vi "SYST_UPR_FPAN_STAT.vi"(0 "VISA IN":refnum<visa-resource-name>, 5 "error in":errorcluster, 7 "Preset":bool) -> (14 "VISA Out":refnum<visa-resource-name>, 19 "error out":errorcluster)   [LabVIEW 2018, in "PNA-X.lvlib"]
doc: "SYSTem:UPReset:FPANel[:STATe] <bool> \n(Read-Write) 'Checks' and 'clears' the enable box on the User Preset dialog box. This only affects \nsubsequent Presets from the front panel user interface. \nRegardless of the state of the User Preset Enable checkbox, the SYST:PRESet command will always \npreset the PNA to the factory preset settings, and SYST:UPReset will always perform a User Preset. \nParameters \n<bool> Front Panel User Preset State. Choose from: \n0 User Preset OFF \n1 User Preset ON \nExamples SYST:UPR:FPAN 1 \nsystem:upreset:fpanel:state 0 \nQuery Syntax SYSTem:UPREset:FPANel[:STATe]? \nReturn Type Boolean \nDefault 0 \n1880"
uses:
  PNA-X.lvlib
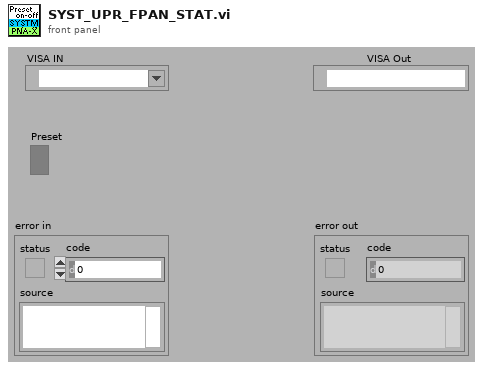
[diagram p1: front panel]
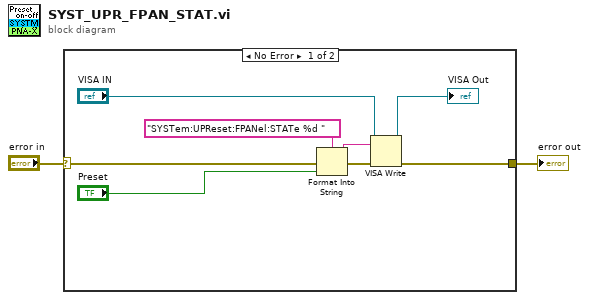
[diagram p0: block diagram]
diagram:
  n1 = case shown="No Error" "error in" {
    selector: "error in" -> [w10 w11]
    tunnel: [w5 w11] -> w1
    frame No Error {
      n2 = Format Into String(format string="SYSTem:UPReset:FPANel:STATe %d " ("Cmdline"), error in=w10, "Preset") -> (resulting string=w8:string, error out=w9:errorcluster)  [unwired: 1 in]
      n3 = VISA Write(VISA resource name="VISA IN", write buffer=w8, error in (no error)=w9) -> (VISA resource name out=→"VISA Out":refnum<visa-resource-name>, error out=w5:errorcluster)  [unwired: 1 out]
    }
    frame Error {
    }
  }
  "error out" <- w1
